vi "libssh2_session_set_last_error.vi"(8 "error in (no error)":errorcluster, 9 "error message":string, 10 "error code":i32, 11 "session":T1) -> (0 "error out":errorcluster)   [LabVIEW 2013, in "libssh2.lvlib"]
doc: "Set the last error code and error message for a session."
uses:
  libssh2.lvlib
  Session Refnum.ctl
  Not A Session.vi
  <vilib>/Utility/error.llb/Error Cluster From Error Code.vi
  Global Settings.vi
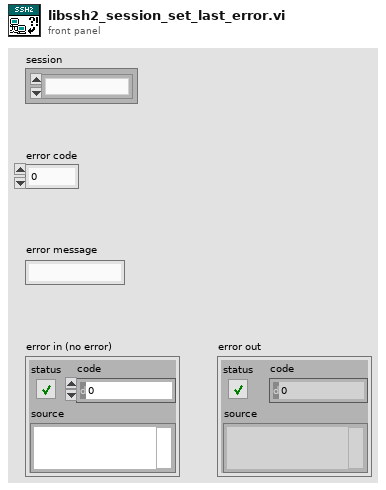
[diagram p1: front panel]
types:
  T1 = typedef "libssh2.lvlib/Session Refnum.ctl" = refnum<k1>
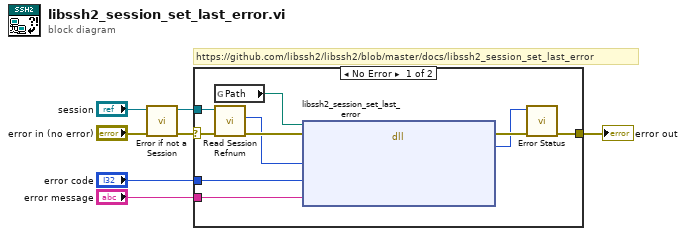
[diagram p0: block diagram]
diagram:
  # "https://github.com/libssh2/libssh2/blob/master/docs/libssh2_session_set_last_error"
  n1 = call "Error if not a Session.vi"("error in (no error)"="error in (no error)", "session"="session") -> ("error out"=w5:errorcluster, "session out"=w3:T1)  [unwired: 8 in]
  n2 = case shown="No Error" w5 {
    selector: w5 -> [w16 w18]
    tunnel: [w9 w18] -> w7
    tunnel: w3 -> [w15 _]
    tunnel: "error code" -> [w11 _]
    tunnel: "error message" -> [w10 _]
    frame No Error {
      n3 = global read "Global Settings.vi" "Path"() -> (w12:path)
      n4 = call "Read Session Refnum.vi"("error in (no error)"=w16, "session"=w15) -> ("error out"=w14:errorcluster, "LIBSSH2_SESSION*"=w13:u64)  [unwired: 5 in, 3 out]
      n5 = dll-call lib="?" fn="libssh2_session_set_last_error"(path in=w12, error in=w14, "session"=w13, "errcode"=w11, "errmsg"=w10) -> (error out=w17:errorcluster, "return value"=w8:i32)  [unwired: 4 in, 1 out]
      n6 = call "Error Status.vi"("error in (no error)"=w17, "return value"=w8) -> ("error out"=w9:errorcluster)  [unwired: 8 in, 1 out]
    }
    frame Error {
    }
  }
  "error out" <- w7
